vi "get laser on.vi"(8 "error in (no error)":errorcluster, 11 "Cobolt in":refnum<class "Cobolt.lvclass">) -> (0 "error out":errorcluster, 3 "Cobolt out":refnum<class "Cobolt.lvclass">)   [LabVIEW 2012, in "Cobolt.lvclass"]
uses:
  Cobolt.lvclass
  CoboltLaserDrivers_Public_LV2012/CoboltLaser_Controls/ExpectedResponseType.ctl
  Cobolt.lvclass/Cobolt.ctl
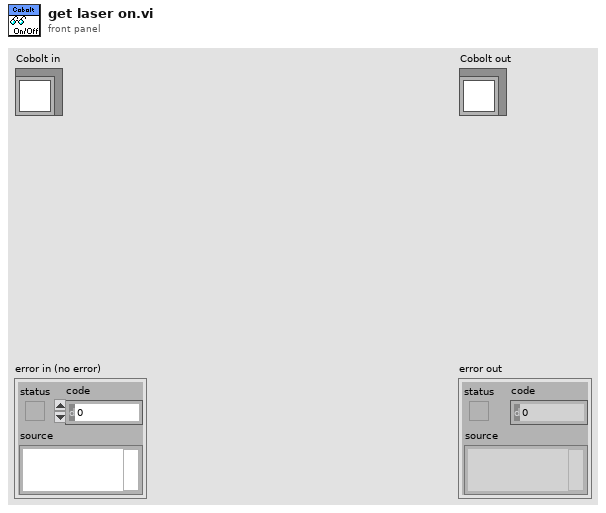
[diagram p1: front panel]
types:
  T1 = typedef "Cobolt.lvclass/ExpectedResponseType.ctl" = u16
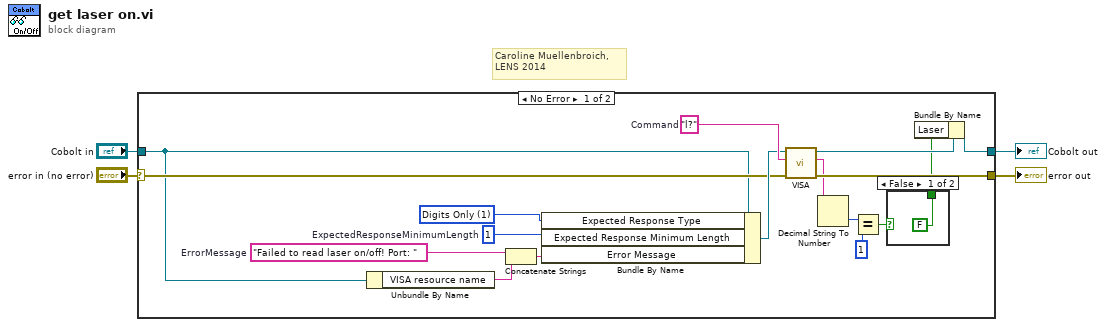
[diagram p0: block diagram]
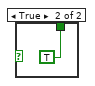
[diagram p2: hidden frame]
diagram:
  # "Caroline Muellenbroich, \nLENS 2014"
  n1 = case shown="No Error" "error in (no error)" {
    selector: "error in (no error)" -> [w13 w25]
    tunnel: [w12 w25] -> w3
    tunnel: [w10 w24] -> w1
    tunnel: "Cobolt in" -> [w11 w24]
    frame No Error {
      w14 = T1 1 items=["Any", "Digits Only", "Non-Digits Only"] ("ExpectedResponseType")
      w18 = 1  # ExpectedResponseMinimumLength
      w16 = "Failed to read laser on/off! Port: "  # ErrorMessage
      w20 = "l?"  # Command
      n2 = Unbundle By Name(w11) -> ("VISA resource name"=w17:string)
      n3 = Concatenate Strings(w16, w17) -> (w15:string)
      n4 = Bundle By Name(cluster=w11, "Expected Response Type"=w14, "Expected Response Minimum Length"=w18, "Error Message"=w15) -> (w19:refnum<class "Cobolt.lvclass">)
      n5 = call-dynamic "VISA.vi"("error in (no error)"=w13, "string to write"=w20, "Cobolt in"=w19) -> ("error out"=w12:errorcluster, "buffer out"=w7:string, "Cobolt out"=w21:refnum<class "Cobolt.lvclass">)  [unwired: 6 in]
      n6 = Decimal String To Number(string=w7) -> (number=w8:i32)  [unwired: 2 in, 1 out]
      n7 = Equal?(x=w8, y=1) -> (x = y?=w6:bool)
      n8 = case shown="False" w6 {
        tunnel: [FALSE TRUE] -> w5
        frame False {
        }
        frame True {
        }
      }
      n9 = Bundle By Name(cluster=w21, "Laser"=w5) -> (w10:refnum<class "Cobolt.lvclass">)
    }
    frame Error {
    }
  }
  "error out" <- w3
  "Cobolt out" <- w1
